vi "DoCreate.vi"(8 "ErrorIn":errorcluster, 11 "YActorIn":refnum<class "YActor.lvclass">) -> (0 "ErrorOut":errorcluster, 3 "YActorOut":refnum<class "YActor.lvclass">)   [LabVIEW 2021, in "YActor.lvclass"]
uses:
  YActor.lvclass
  YActor.lvclass/YActor.ctl
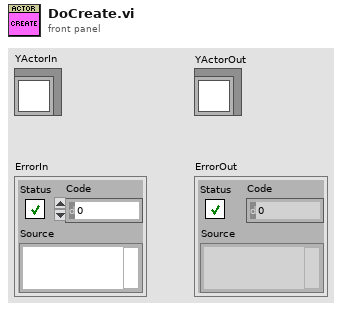
[diagram p1: front panel]
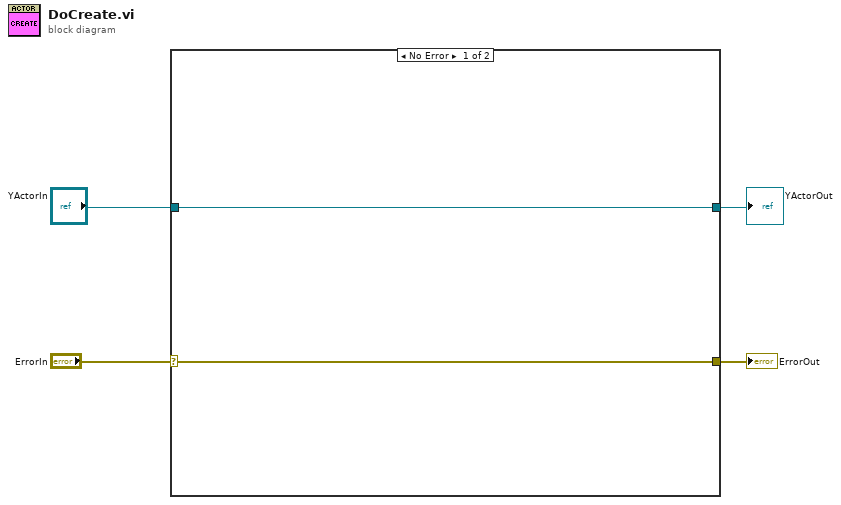
[diagram p0: block diagram]
diagram:
  n1 = case shown="No Error" "ErrorIn" {
    selector: "ErrorIn" -> [w6 w8]
    tunnel: [w6 w8] -> w3
    tunnel: "YActorIn" -> [w5 w7]
    tunnel: [w5 w7] -> w1
    frame No Error {
    }
    frame Error {
    }
  }
  "ErrorOut" <- w3
  "YActorOut" <- w1
